vi "Acquistion-Loop.vi"(8 "error in":errorcluster, 10 "Unprocessed Data":refnum<queue>, 11 "Message Queues":T1) -> (0 "error out":errorcluster)   [LabVIEW 2024]
uses:
  support/Message Queue/All Message Queues.ctl
  support/Message Queue/Message Cluster.ctl
  support/Control/Waveform Data Constant.ctl
  Acquisition State.ctl
  support/Control/DAQmx Container.ctl
  Configuration/DAQmx Configuration.ctl
  Globals.vi
  <vilib>/ErrorRing/Error Ring.xnode
  support/Message Queue/Message Queue.lvlib
panel:
  out "Loop-1 Iteration Counter":i32
  out "Loop-1 Iteration Clock (ms)":u32
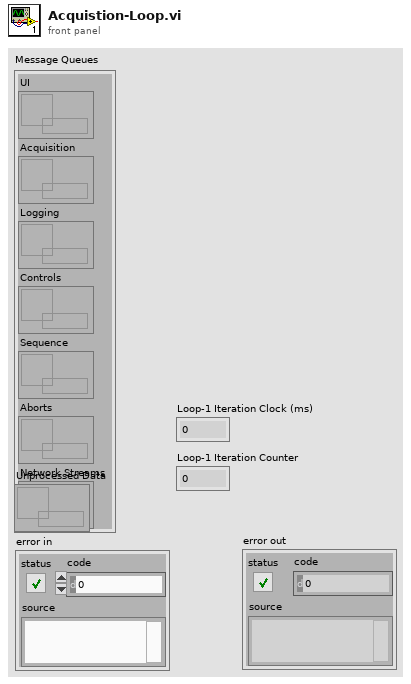
[diagram p1: front panel]
types:
  T1 = typedef "Message Queue.lvlib/All Message Queues.ctl" = cluster{"UI":refnum<queue>, "Acquisition":refnum<queue>, "Logging":refnum<queue>, "Controls":refnum<queue>, "Sequence":refnum<queue>, "Aborts":refnum<queue>, "Network Streams":refnum<queue>}
  T2 = typedef "DAQmx Configuration.ctl" = cluster{"ai DAQmx Cluster":cluster{"ai PXIe Task Name":string[], "input terminal configuration":i32[]}, "bc DAQmx Cluster":cluster{"bc PXIe Task Name":string[], "Scaling Information":cluster{"first electrical value":dbl, "second electrical value":dbl, "electrical units":i32, "first physical value":dbl, "second physical value":dbl, "physical units":i32}[], "Bridge Information":cluster{"bridge configuration":i32, "voltage excitation source":i32, "voltage excitation value":dbl, "nominal bridge resistance":dbl}[]}, "tc DAQmx Cluster":cluster{"tc PXIe Task Name":string[], "Thermocouple Type":i32[], "Units":i32[]}, "di DAQmx Cluster":cluster{"di PXIe Task Name":string[]}, "do DAQmx Cluster":cluster{"do PXIe Task Name":string[]}, "ao DAQmx Cluster":cluster{"ao PXIe Task Name":string[]}}
  T3 = typedef "DAQmx Container.ctl" = cluster{"DAQmx Analog In":refnum<k21>, "DAQmx Digital In":refnum<k21>, "DAQmx Digital Out":refnum<k21>, "DAQmx Analog Out":refnum<k21>, "DAQmx 6343":refnum<k21>, "DAQmx IG-Sense":refnum<k21>, "DAQmx Thermo":refnum<k21>, "DAQmx Bridge":refnum<k21>, "DAQmx Trigger":refnum<k21>}
  T4 = typedef "Acquisition State.ctl" = enum16{"Idle", "Acquiring"}
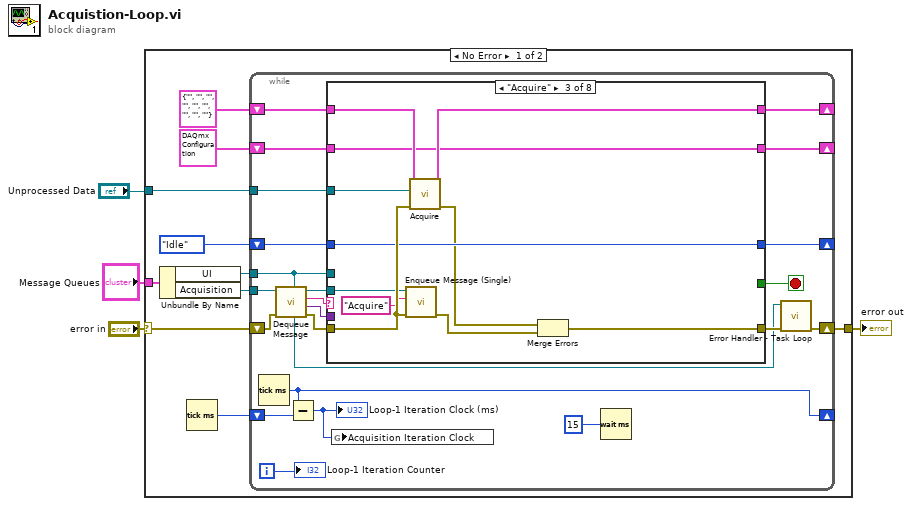
[diagram p0: block diagram]
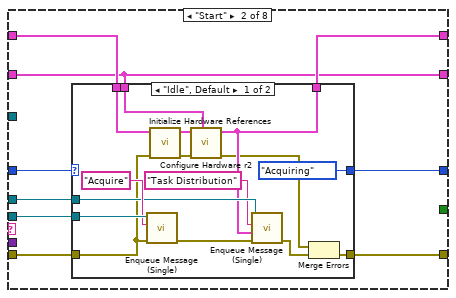
[diagram p3: hidden frame]
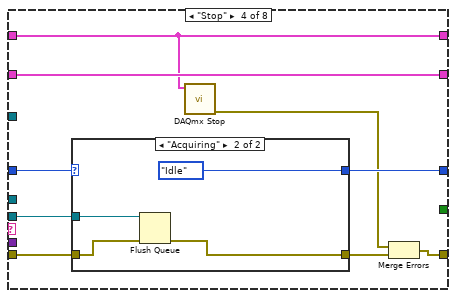
[diagram p5: hidden frame]
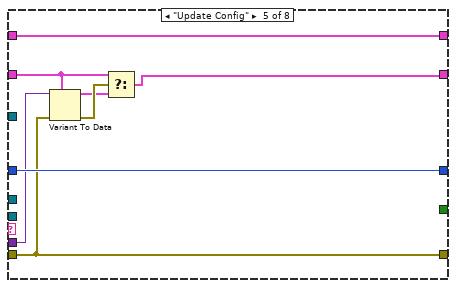
[diagram p7: hidden frame]
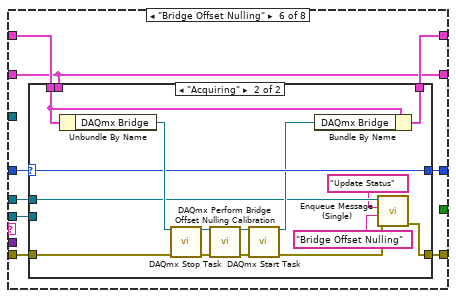
[diagram p8: hidden frame]
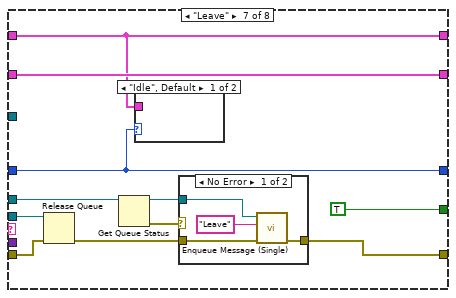
[diagram p10: hidden frame]
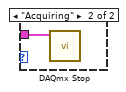
[diagram p12: hidden frame]
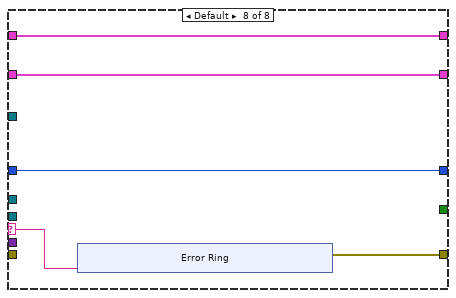
[diagram p13: hidden frame]
diagram:
  n1 = case shown="No Error" "error in" {
    selector: "error in" -> [w14 w156]
    tunnel: "Message Queues" -> [w11 _]
    tunnel: "Unprocessed Data" -> [w12 _]
    tunnel: [w13 w156] -> w2
    frame No Error {
      n2 = Unbundle By Name(w11) -> ("UI"=w9:refnum<queue>, "Acquisition"=w10:refnum<queue>)
      n3 = Tick Count (ms)() -> (millisecond timer value=w7:u32)
      n4 = while {
        shift-right: [w28] -> w13
        shift-left: w14 -> [w36]
        tunnel: w12 -> [w30]
        tunnel: w10 -> [w35]
        tunnel: w9 -> [w26]
        shift-right: [w25] -> _
        shift-left: T2 {"ai DAQmx Cluster"={"ai PXIe Task Name"=[], "input terminal configuration"=[]}, "bc DAQmx Cluster"={"bc PXIe Task Name"=[], "Scaling Information"=[], "Bridge Information"=[]}, "tc DAQmx Cluster"={"tc PXIe Task Name"=[], "Thermocouple Type"=[], "Units"=[]}, "di DAQmx Cluster"={"di PXIe Task Name"=[]}, "do DAQmx Cluster"={"do PXIe Task Name"=[]}, "ao DAQmx Cluster"={"ao PXIe Task Name"=[]}} ("DAQmx Cluster") -> [w29]
        shift-right: [w23] -> _
        shift-left: Acquisition_State."Idle" ("Acquisition State") -> [w24]
        shift-right: [w20] -> _
        shift-left: w7 -> [w21]
        shift-right: [w16] -> _
        shift-left: T3 {"DAQmx Analog In"="", "DAQmx Digital In"="", "DAQmx Digital Out"="", "DAQmx Analog Out"="", "DAQmx 6343"="", "DAQmx IG-Sense"="", "DAQmx Thermo"="", "DAQmx Bridge"="", "DAQmx Trigger"=""} ("DAQmx Container") -> [w17]
        i -> [w19]
        stop <- w22 stop-if-true
        n5 = Tick Count (ms)() -> (millisecond timer value=w20:u32)
        n6 = call "Dequeue Message.vi"("error in (no error)"=w36, "Message Queue"=w35) -> ("error out"=w31:errorcluster, "Message Data"=w32:variant, "Message"=w33:string, "dup Message Queue"=w34:refnum<queue>)  [unwired: 6 in]
        n7 = Subtract(x=w20, y=w21) -> (x-y=w15:u32)
        "Loop-1 Iteration Clock (ms)" <- w15
        n8 = case shown="\"Acquire\"" w33 {
          selector: w33 -> [_ _ _ _ _ _ _ w147]
          tunnel: w34 -> [_ w46 w76 w85 _ w107 w139 _]
          tunnel: w32 -> [_ _ _ _ w100 _ _ _]
          tunnel: w31 -> [w40 w47 w78 w84 w99 w108 w138 _]
          tunnel: w26 -> [_ w42 _ _ _ w103 w133 _]
          tunnel: w30 -> [_ _ w71 _ _ _ _ _]
          tunnel: w29 -> [w39 w41 w68 w82 w97 w102 w137 w149]
          tunnel: [w40 w45 w74 w80 w99 w106 w134 w148] -> w27
          tunnel: [w39 w41 w68 w82 w95 w102 w137 w149] -> w25
          tunnel: w24 -> [w38 w49 w77 w87 w101 w110 w135 w150]
          tunnel: [w38 w48 w77 w86 w101 w109 w135 w150] -> w23
          tunnel: [_ _ _ _ _ _ TRUE _] -> w22
          tunnel: w17 -> [w37 w44 w70 w81 w94 w105 w136 w146]
          tunnel: [w37 w43 w69 w81 w94 w104 w136 w146] -> w16
          frame "Initialize" {
          }
          frame "Start" {
            n9 = case shown="\"Idle\", Default" w49 {
              selector: w49 -> [_ w66]
              tunnel: [Acquisition_State."Acquiring" ("Acquisition State") w66] -> w48
              tunnel: w47 -> [w55 w67]
              tunnel: w46 -> [w63 _]
              tunnel: [w61 w67] -> w45
              tunnel: w44 -> [w56 w65]
              tunnel: [w52 w65] -> w43
              tunnel: w42 -> [w59 _]
              tunnel: w41 -> [w50 _]
              frame "Idle", Default {
                n10 = call "Enqueue Message (Single).vi"("error in (no error)"=w55, "Message"="Acquire", "Message Queue"=w63) -> ("error out"=w60:errorcluster)  [unwired: 7 in, 1 out]
                n11 = call "Initialize Hardware References.vi"("error in (no error)"=w55, "DAQmx Container In"=w56) -> ("error out"=w54:errorcluster, "DAQmx Container Out"=w53:T3)  [unwired: 8 in]
                n12 = call "Configure Hardware r2.vi"("DAQmx Cluster In"=w50, "error in (no error)"=w54, "DAQmx Container In"=w53) -> ("error out"=w51:errorcluster, "DAQmx Container Out"=w52:T3)  [unwired: 7 in]
                n13 = call "Enqueue Message (Single).vi"("error in (no error)"=w60, "Message Data"=w52, "Message"="Task Distribution", "Message Queue"=w59) -> ("error out"=w58:errorcluster)  [unwired: 6 in, 1 out]
                n14 = Merge Errors(w51, w58) -> (w61:errorcluster)
              }
              frame "Acquiring" {
              }
            }
          }
          frame "Acquire" {
            n15 = call "Enqueue Message (Single).vi"("error in (no error)"=w78, "Message"="Acquire", "Message Queue"=w76) -> ("error out"=w73:errorcluster)  [unwired: 7 in, 1 out]
            n16 = call "Acquire.vi"("DAQmx Container In"=w70, "Unprocessed Data"=w71, "error in (no error)"=w78) -> ("DAQmx Container Out"=w69:T3, "error out"=w72:errorcluster)  [unwired: 6 in]
            n17 = Merge Errors(w72, w73) -> (w74:errorcluster)
          }
          frame "Stop" {
            n18 = case shown="\"Acquiring\"" w87 {
              selector: w87 -> [w89 _]
              tunnel: [w89 Acquisition_State."Idle" ("Acquisition State")] -> w86
              tunnel: w85 -> [_ w92]
              tunnel: w84 -> [w88 w91]
              tunnel: [w88 w90] -> w83
              frame "Idle", Default {
              }
              frame "Acquiring" {
                n19 = Flush Queue(queue=w92, error in (no error)=w91) -> (error out=w90:errorcluster)  [unwired: 2 out]
              }
            }
            n20 = call "DAQmx Stop.vi"("DAQmx Container"=w81) -> ("error out"=w79:errorcluster)  [unwired: 10 in]
            n21 = Merge Errors(w79, w83) -> (w80:errorcluster)
          }
          frame "Update Config" {
            n22 = Variant To Data(error in=w99, type=w97, Variant=w100) -> (data=w96:T2, error out=w98:errorcluster)
            n23 = Select(t=w97, s=w98, f=w96) -> (s? t:f=w95:T2)
          }
          frame "Bridge Offset Nulling" {
            n24 = case shown="\"Acquiring\"" w110 {
              selector: w110 -> [w112 w124]
              tunnel: [w112 w124] -> w109
              tunnel: w108 -> [w113 w118]
              tunnel: w107 -> [_ _]
              tunnel: [w113 w115] -> w106
              tunnel: w105 -> [w111 w126]
              tunnel: [w111 w127] -> w104
              tunnel: w103 -> [_ w119]
              tunnel: w102 -> [_ _]
              frame "Idle", Default {
              }
              frame "Acquiring" {
                n25 = Unbundle By Name(w126) -> ("DAQmx Bridge"=w128:refnum<k21>)
                n26 = call <vilib>:"DAQmx Stop Task.vi"("task/channels in"=w128, "error in"=w118) -> ("task out"=w123:refnum<k21>, "error out"=w122:errorcluster)  [unwired: 12 in]
                n27 = call <vilib>:"DAQmx Perform Bridge Offset Nulling Calibration.vi"("task/channels in"=w123, "error in"=w122) -> ("task out"=w125:refnum<k21>, "error out"=w120:errorcluster)  [unwired: 12 in]
                n28 = call <vilib>:"DAQmx Start Task.vi"("task/channels in"=w125, "error in"=w120) -> ("task out"=w121:refnum<k21>, "error out"=w114:errorcluster)  [unwired: 12 in]
                n29 = Bundle By Name(cluster=w126, "DAQmx Bridge"=w121) -> (w127:T3)
                n30 = call "Enqueue Message (Single).vi"("error in (no error)"=w114, "Message Data"="Bridge Offset Nulling", "Message"="Update Status", "Message Queue"=w119) -> ("error out"=w115:errorcluster)  [unwired: 6 in, 1 out]
              }
            }
          }
          frame "Leave" {
            n31 = Release Queue(queue=w139, error in (no error)=w138) -> (error out=w130:errorcluster)  [unwired: 1 in, 2 out]
            n32 = Get Queue Status(queue=w133) -> (queue out=w131:refnum<queue>, error out=w129:errorcluster)  [unwired: 2 in, 6 out]
            n33 = case shown="\"Idle\", Default" w135 {
              tunnel: w136 -> [_ w145]
              frame "Idle", Default {
              }
              frame "Acquiring" {
                n34 = call "DAQmx Stop.vi"("DAQmx Container"=w145) -> ()  [unwired: 10 in, 1 out]
              }
            }
            n35 = case shown="No Error" w129 {
              tunnel: [w143 w144] -> w134
              tunnel: w131 -> [w141 _]
              tunnel: w130 -> [w140 w144]
              frame No Error {
                n36 = call "Enqueue Message (Single).vi"("error in (no error)"=w140, "Message"="Leave", "Message Queue"=w141) -> ("error out"=w143:errorcluster)  [unwired: 7 in, 1 out]
              }
              frame Error {
              }
            }
          }
          frame Default {
            n37 = xnode "Error Ring"("parameter 0"=w147) -> ("error out"=w148:errorcluster)
          }
        }
        n38 = global write "Globals.vi" "Acquisition Iteration Clock"(w15) -> ()
        n39 = Wait (ms)(milliseconds to wait=u32 15) -> ()  [unwired: 1 out]
        n40 = call "Error Handler - Task Loop.vi"("error in (no error)"=w27, "Message Queue"=w26) -> ("dup error in"=w28:errorcluster)  [unwired: 8 in, 1 out]
        "Loop-1 Iteration Counter" <- w19
      }
    }
    frame Error {
    }
  }
  "error out" <- w2
